vi "call include vi script.vi"(8 "error in (no error)":errorcluster, 11 "state cluster":T1) -> (0 "error out":errorcluster)   [LabVIEW 2013, in "Standard Editor.lvlib"]
uses:
  Standard Editor.lvlib
  Controls/StateCluster.ctl
  Configuration Editor/Classes/SystemConfigRepo/SystemConfigRepo.lvclass
  Configuration Editor/Classes/Systems/Systems.lvclass
  SplashScreen/splash screen.ctl
  SplashScreen/notifier data.ctl
  <vilib>/NI/Configuration Framework/Node/StandardEvents.ctl
  <vilib>/NI/Configuration Framework/Node/UserEventRef.ctl
  <vilib>/NI/Configuration Framework/Controls/EventCluster.ctl
  <vilib>/NI/Configuration Framework/Node/NodeChangeEvent.ctl
  <vilib>/NI/Configuration Framework/Node/NodeRef.ctl
  <vilib>/NI/Configuration Framework/Node/NISE_CEF_Node.lvclass
  <vilib>/NI/Configuration Framework/Node/CacheState.ctl
  <vilib>/NI/Configuration Framework/Node/RefreshUIEvent.ctl
  <vilib>/NI/Configuration Framework/Node/StopEvent.ctl
  <vilib>/NI/Configuration Framework/glyph manager/glyph manager.ctl
  <vilib>/picture/picture.llb/imagedata.ctl
  Framework Configuration Classes/class cache/PL_class cache.lvlib
  <vilib>/NI/Configuration Framework/NISE_CEF_TreeControl.lvlib
  SplashScreen/Standard Editor splash screen.lvlib
  <vilib>/NI/Configuration Framework/glyph manager/glyph manager.lvlib
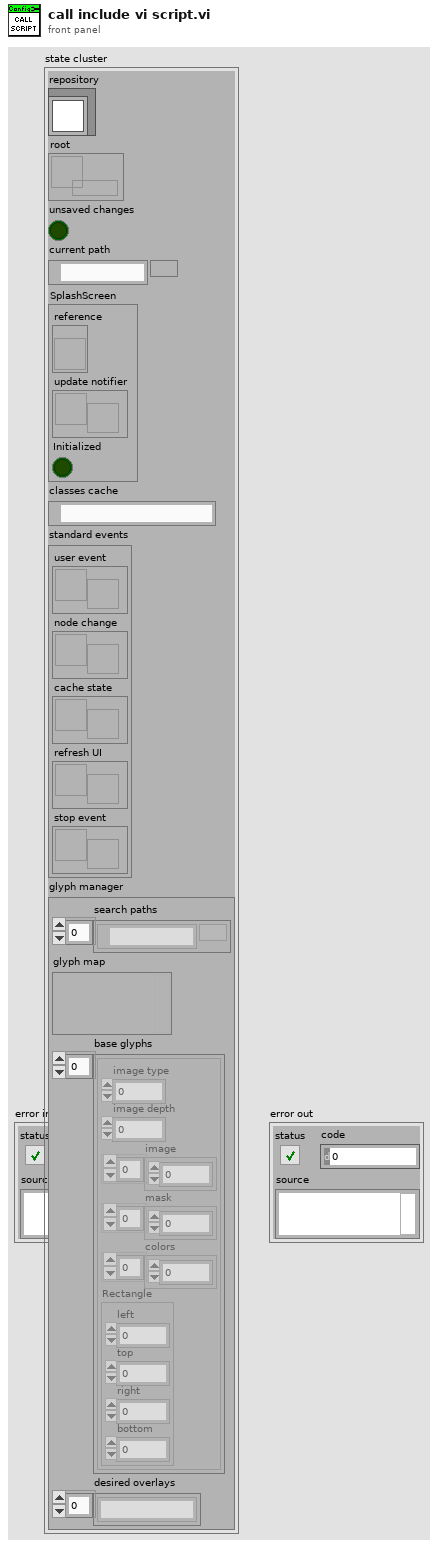
[diagram p1: front panel]
types:
  T1 = typedef "Standard Editor.lvlib/StateCluster.ctl" = cluster{"repository":refnum<class "SystemConfigRepo.lvclass">, "root":refnum<data-value>, "unsaved changes":bool, "current path":path, "SplashScreen":T2, "classes cache":path, "standard events":T3, "glyph manager":T9}
  T2 = typedef "Standard Editor splash screen.lvlib/splash screen.ctl" = cluster{"reference":refnum<vi>, "update notifier":refnum<notifier>, "Initialized":bool}
  T3 = typedef "NISE_CEF_Node.lvclass/StandardEvents.ctl" = cluster{"user event":T4, "node change":T5, "cache state":T6, "refresh UI":T7, "stop event":T8}
  T4 = typedef "NISE_CEF_Node.lvclass/UserEventRef.ctl" = refnum<user-event>
  T5 = typedef "NISE_CEF_Node.lvclass/NodeChangeEvent.ctl" = refnum<user-event>
  T6 = typedef "NISE_CEF_Node.lvclass/CacheState.ctl" = refnum<user-event>
  T7 = typedef "NISE_CEF_Node.lvclass/RefreshUIEvent.ctl" = refnum<user-event>
  T8 = typedef "NISE_CEF_Node.lvclass/StopEvent.ctl" = refnum<user-event>
  T9 = typedef "glyph manager.lvlib/glyph manager.ctl" = cluster{"search paths":path[], "glyph map":variant, "base glyphs":T10[], "desired overlays":string[]}
  T10 = typedef "imagedata.ctl" = cluster{"image type":i32, "image depth":i32, "image":u8[], "mask":u8[], "colors":u32[], "Rectangle":cluster{"left":i16, "top":i16, "right":i16, "bottom":i16}}
  T11 = typedef "PL_class cache.lvlib/cache definition.ctl" = cluster{"configuration":T12, "class cache data":T13}
  T12 = typedef "PL_class cache.lvlib/cache search configuration.ctl" = cluster{"Search Paths":path[], "Folders to Exclude":string[], "full class list":path[]}
  T13 = typedef "PL_class cache.lvlib/cached class information.ctl" = cluster{"targets":T14[], "engines":T15[], "modules":T15[], "ignored class list":path[]}
  T14 = typedef "PL_class cache.lvlib/target class metadata.ctl" = cluster{"file name":string, "fully qualified name":string, "menu display name":string, "configuration class name":string}
  T15 = typedef "PL_class cache.lvlib/class metadata.ctl" = cluster{"file name":string, "fully qualified name":string, "menu display name":string, "configuration class":string, "instances allowed":i32, "supported targets":T16[]}
  T16 = typedef "TBM configuration.lvclass/Target Types.ctl" = enum16{"Windows", "Mac", "Linux", "Linux RT ARM", "VxWorks", "Pharlap", "Other", "Linux RT x64"}
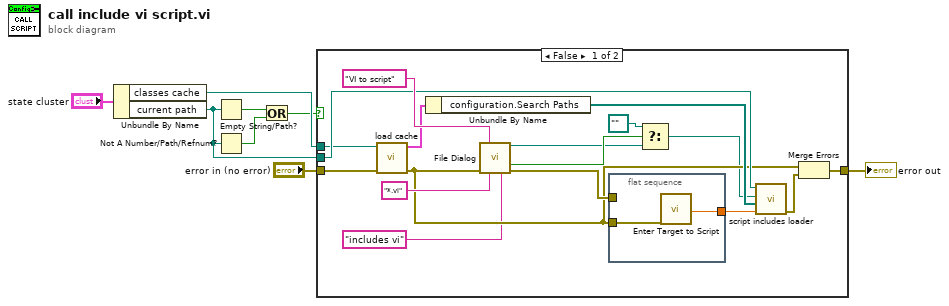
[diagram p0: block diagram]
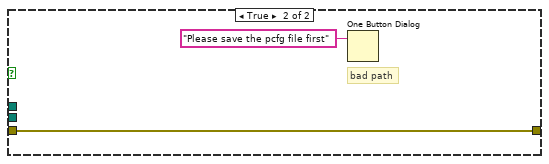
[diagram p2: hidden frame]
diagram:
  n1 = Unbundle By Name("state cluster") -> ("classes cache"=w6:path, "current path"=w5:path)
  n2 = Empty String/Path?(string/path=w5) -> (empty?=w3:bool)
  n3 = Not A Number/Path/Refnum?(number/path/refnum=w5) -> (NaN/Path/Refnum?=w2:bool)
  n4 = Or(x=w3, y=w2) -> (x .or. y?=w4:bool)
  n5 = case shown="False" w4 {
    tunnel: w5 -> [w22 _]
    tunnel: w6 -> [w19 _]
    tunnel: "error in (no error)" -> [w18 w28]
    tunnel: [w16 w28] -> w8
    frame False {
      n6 = call "load cache.vi"("error in"=w18, "cache path"=w19) -> ("error out"=w14:errorcluster, "cache"=w23:T11)  [unwired: 8 in]
      n7 = Unbundle By Name(w23) -> ("configuration.Search Paths"=w21:path[])
      n8 = call "File Dialog"("prompt"="VI to script", "error in"=w14, "pattern (all files)"="*.vi", "pattern label"="includes vi") -> ("selected path"=w11:path, "cancelled"=w12:bool, "error out"=w15:errorcluster)  [unwired: 8 in, 1 out]
      n9 = flat-sequence {
        tunnel: [w27] -> w20
        tunnel: w15 -> [_]
        tunnel: w14 -> [w26]
        frame #0 {
          n10 = call "Enter Target to Script"("error in (no error)"=w26) -> ("Target Number (0)"=w27:dbl)  [unwired: 16 in, 2 out]
        }
      }
      n11 = Select(t=path "", s=w12, f=w11) -> (s? t:f=w13:path)
      n12 = call "script includes loader.vi"("target"=w20, "Plugin Search Paths"=w21, "vi path (blank=new)"=w13, "pcfg file path"=w22) -> ("error out"=w17:errorcluster)  [unwired: 7 in]
      n13 = Merge Errors(w14, w17) -> (w16:errorcluster)
    }
    frame True {
      # "bad path"
      n14 = One Button Dialog(message="Please save the pcfg file first") -> ()  [unwired: 1 in, 1 out]
    }
  }
  "error out" <- w8
